vi "version.vi"(7 "LabVIEW Web Service Request":refnum<class "Web Request.lvclass">) -> ()   [LabVIEW 2015]
uses:
  <vilib>/wsapi/Web Request.lvclass
  lv-hello-world/lv-hello-world.lvlib
panel:
  # "Use the Web Service Request input terminal to call the VIs on the Web Services palette. Do not remove it from the connector pane unless you don't need access to the palette."
  # "Each additional control wired to the connector pane will be available as an input in the URL. To include an indicator in terminal-mode output (the default setting), it must also be wired to the connector pane."
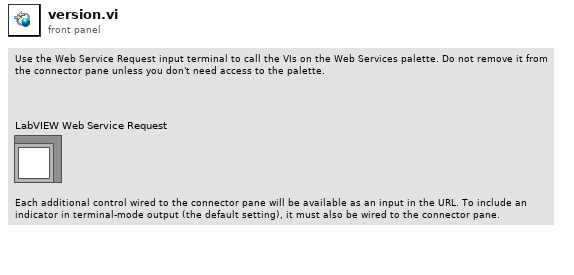
[diagram p1: front panel]
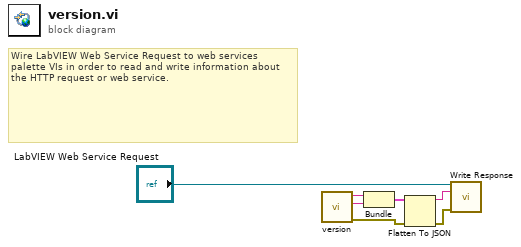
[diagram p0: block diagram]
diagram:
  # "Wire LabVIEW Web Service Request to web services palette VIs in order to read and write information about the HTTP request or web service."
  n1 = call "version.vi"() -> ("error out"=w3:errorcluster, "commit"=w5:string, "version"=w6:string)  [unwired: 9 in]
  n2 = Bundle("version"=w6, "commit"=w5) -> (w4:cluster{"version":string, "commit":string})  [unwired: 1 in]
  n3 = Flatten To JSON(anything=w4, error in (no error)=w3) -> (JSON string=w2:string, 11:w1:errorcluster)  [unwired: 1 in]
  n4 = call <vilib>:"Write Response.vi"("LabVIEW Web Service Request"="LabVIEW Web Service Request", "response string"=w2, "error in (no error)"=w1) -> ()  [unwired: 11 in, 2 out]
